vi "ini_test.vi"() -> ()   [LabVIEW 2010]
uses:
  <vilib>/Utility/config.llb/NI_LVConfig.lvlib
panel:
  out "element":string
  out "list":string[](array[string])
  out "default":i32
  in  "section":string="param1"
  in  "par_val":string="Описание работы"
  out "error out":errorcluster
  in  "error in (no error)":errorcluster
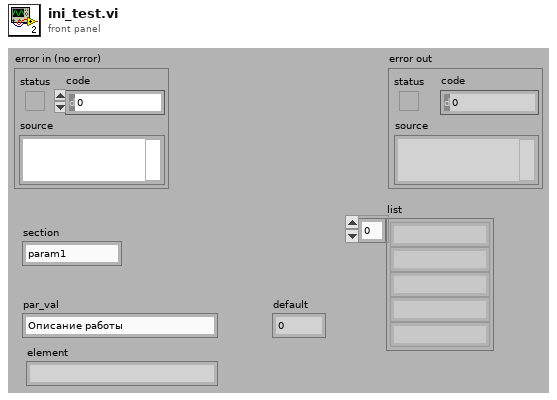
[diagram p1: front panel]
types:
  T1 = typedef "NI_LVConfig.lvlib/Config Data RefNum.ctl" = refnum<k1>
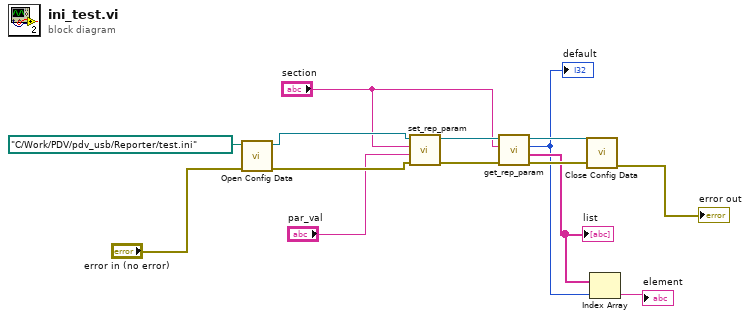
[diagram p0: block diagram]
diagram:
  n1 = call <vilib>:"Open Config Data.vi"("error in (no error)"="error in (no error)", "configuration file path"=path "C:/Work/PDV/pdv_usb/Reporter/test.ini") -> ("error out"=w13:errorcluster, "refnum"=w14:T1)  [unwired: 7 in, 1 out]
  n2 = call "set_rep_param.vi"("error in (no error)"=w13, "par_val"="par_val", "param_name"="section", "refnum"=w14) -> ("error out"=w8:errorcluster, "refnum out"=w6:T1)  [unwired: 2 in]
  n3 = call "get_rep_param.vi"("error in (no error)"=w8, "param_name"="section", "refnum"=w6) -> ("error out"=w7:errorcluster, "list"=w3:string[], "default"=w2:i32, "refnum out"=w5:T1)  [unwired: 1 in]
  "default" <- w2
  "list" <- w3
  n4 = call <vilib>:"Close Config Data.vi"("error in (no error)"=w7, "refnum"=w5) -> ("error out"=→"error out":errorcluster)  [unwired: 8 in, 1 out]
  n5 = Index Array(array=w3, index=w2) -> (element=→"element":string)
